vi "Test NT Server.vi"() -> ()   [LabVIEW 2015]
panel:
  out "Connection Count":i32
  out "Connected":bool
  in  "stop":bool
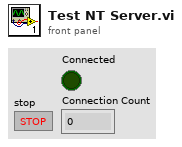
[diagram p1: front panel]
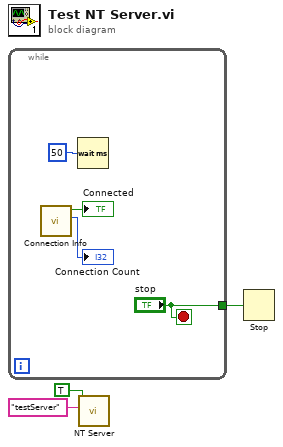
[diagram p0: block diagram]
diagram:
  n1 = while {
    tunnel: ["stop"] -> w3
    stop <- "stop" stop-if-true
    n2 = call <vilib>:"Connection Info.vi"() -> ("Connection Count"=→"Connection Count":i32, "Connected"=→"Connected":bool)  [unwired: 10 in]
    n3 = Wait (ms)(milliseconds to wait=u32 50) -> ()  [unwired: 1 out]
  }
  n4 = call <vilib>:"NT Server.vi"("Server Name"="testServer", "Enable Read Errors"=TRUE) -> ()  [unwired: 10 in]
  n5 = Stop(stop? (T)=w3) -> ()
